vi "update_ctrl;.vi"() -> ()   [LabVIEW 2015]
panel:
  out "output variable 1":dbl
  in  "Inp1":dbl
  out "output variable 2":dbl
  in  "Inp2":dbl
  in  "OK Button":bool
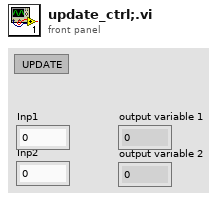
[diagram p1: front panel]
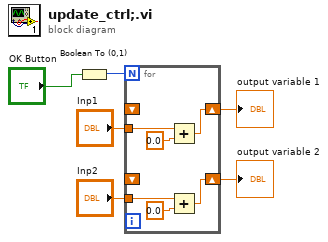
[diagram p0: block diagram]
diagram:
  n1 = Boolean To (0,1)(Boolean="OK Button") -> (0, 1=w5:i16)
  n2 = for {
    N: w5 -> [_]
    tunnel: "Inp2" -> [w11]
    shift-right: [w10] -> w3
    shift-left: _ -> [_]
    tunnel: "Inp1" -> [w8]
    shift-right: [w7] -> w1
    shift-left: _ -> [_]
    n3 = Add(x=w8, y=0.0) -> (x+y=w7:dbl)
    n4 = Add(x=w11, y=0.0) -> (x+y=w10:dbl)
  }
  "output variable 2" <- w3
  "output variable 1" <- w1
